vi "Initialize.vi"(8 "error in (no error)":errorcluster, 9 "ZMQ context":refnum<class "zmq_context.lvclass">, 10 "Name":string, 11 "NewSocket in":refnum<class "NewSocket.lvclass">) -> (0 "error out":errorcluster, 3 "NewSocket out":refnum<class "NewSocket.lvclass">)   [LabVIEW 2018, in "NewSocket.lvclass"]
uses:
  NewSocket.lvclass
  <vilib>/addons/zeromq/zmq_context.lvclass
  NewSocket.lvclass/NewSocket.ctl
  State Machine/CM_State Machine.lvclass
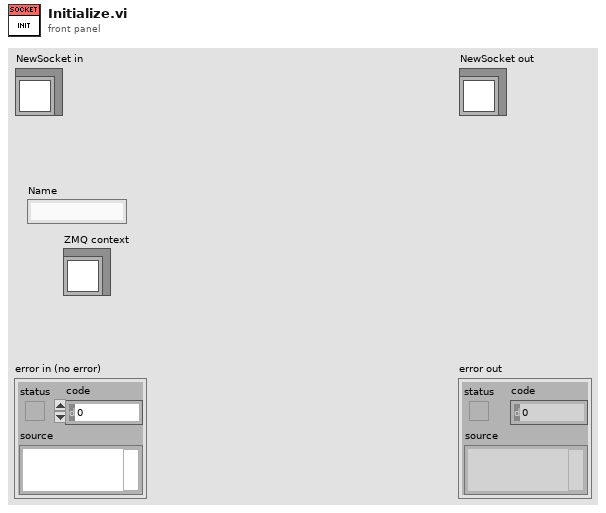
[diagram p1: front panel]
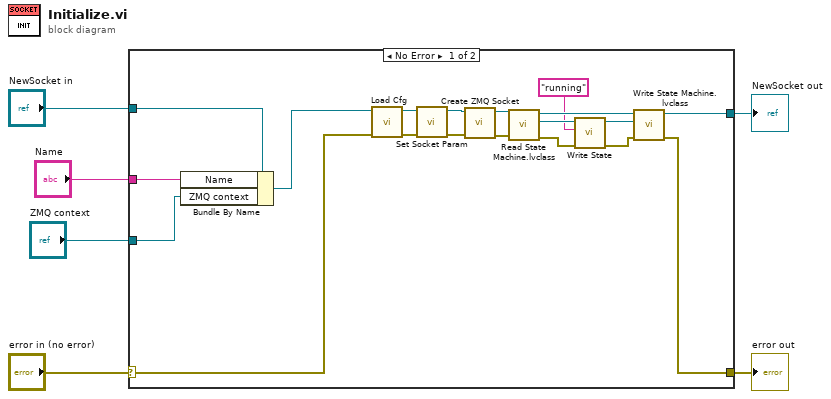
[diagram p0: block diagram]
diagram:
  n1 = case shown="No Error" "error in (no error)" {
    selector: "error in (no error)" -> [w15 w27]
    tunnel: [w9 w27] -> w5
    tunnel: [w17 w26] -> w3
    tunnel: "NewSocket in" -> [w25 w26]
    tunnel: "Name" -> [w8 _]
    tunnel: "ZMQ context" -> [w7 _]
    frame No Error {
      n2 = Bundle By Name(cluster=w25, "Name"=w8, "ZMQ context"=w7) -> (w24:refnum<class "NewSocket.lvclass">)
      n3 = call-dynamic "Load Cfg.vi"("error in (no error)"=w15, "NewSocket in"=w24) -> ("error out"=w14:errorcluster, "NewSocket out"=w23:refnum<class "NewSocket.lvclass">)  [unwired: 8 in]
      n4 = call-dynamic "Set Socket Param.vi"("error in (no error)"=w14, "NewSocket in"=w23) -> ("error out"=w13:errorcluster, "NewSocket out"=w22:refnum<class "NewSocket.lvclass">)  [unwired: 8 in]
      n5 = call-dynamic "Create ZMQ Socket.vi"("error in (no error)"=w13, "NewSocket in"=w22) -> ("error out"=w12:errorcluster, "NewSocket out"=w19:refnum<class "NewSocket.lvclass">)  [unwired: 8 in]
      n6 = call-dynamic "Read State Machine.lvclass.vi"("error in (no error)"=w12, "NewSocket in"=w19) -> ("error out"=w11:errorcluster, "State Machine.lvclass"=w21:refnum<class "CM_State Machine.lvclass">, "NewSocket out"=w18:refnum<class "NewSocket.lvclass">)  [unwired: 7 in]
      n7 = call-dynamic "Write State.vi"("error in (no error)"=w11, "State"="running", "State Machine in"=w21) -> ("error out"=w10:errorcluster, "State Machine out"=w20:refnum<class "CM_State Machine.lvclass">)  [unwired: 7 in]
      n8 = call-dynamic "Write State Machine.lvclass.vi"("error in (no error)"=w10, "State Machine.lvclass"=w20, "NewSocket in"=w18) -> ("error out"=w9:errorcluster, "NewSocket out"=w17:refnum<class "NewSocket.lvclass">)  [unwired: 7 in]
    }
    frame Error {
    }
  }
  "error out" <- w5
  "NewSocket out" <- w3
